vi "Aplicacao_v02.vi"() -> ()   [LabVIEW 2014]
uses:
  LabView_v03/testStateMachineCtr.ctl
  LabView_v03/testMachineCtr.ctl
  <vilib>/Analysis/baseanly.llb/Mean (DBL).vi
  <vilib>/express/express shared/transition.llb/Dynamic To Waveform Array.vi
  <vilib>/express/express signal manip/GetorSetDDTAttributes/Set DDT Attributes/SetT0.vi
  <vilib>/express/express shared/transition.llb/Waveform Array To Dynamic.vi
  <vilib>/express/express signal manip/GetorSetDDTAttributes/Set DDT Attributes/Set DDT Properties.xnode
  <vilib>/Analysis/NI_AALBase.lvlib
panel:
  in  "editSetPathToFile":path
  out "ledForce":bool caption="Célula de Carga"
  out "ledSpeed":bool caption="Velocidade"
  out "ledTempB":bool caption="Temperatura B"
  out "ledTempA":bool caption="Temperatura A"
  out "ledTempRef":bool caption="Referência"
  in  "buttonExit":bool
  in  "buttonStop":bool
  in  "buttonStart":bool
  out "graphForce":dynamicdata(graph)
  in  "editOffsetForce":dbl caption="Tara" min=0.0 max=100.0 step=0.1
  in  "editSetForce":dbl caption="Fator de conversão"
  out "editForce":dbl caption="Força (Kgf)" format="%#_4f"
  out "graphSpeed":dynamicdata(graph)
  in  "editSetSpeed":dbl caption="Fator de conversão"
  out "editSpeed":dbl caption="Velocidade (km/h)" format="%#_4f"
  out "editEngineSpeed":dbl caption="Rotação (RPM)" format="%#_4f"
  in  "buttonMotor":bool
  in  "buttonBrake":bool
  in  "editSetWaitLowerTime":u32 caption="Tempo de espera (s)"
  in  "editSetWaitUpperTime":u32 caption="Tempo de espera (s)"
  in  "editSetNumberOfCycles":u32 caption="Número de ciclos" max=999 step=1 format="%0d"
  in  "editSetLowerLimit":u32 caption="Limite inferior (km/h)"
  in  "editSetUpperLimit":u32 caption="Limite superior (km/h)"
  out "editTempB":dbl caption="Temperatura B (ºC)"
  out "editTempA":dbl caption="Temperatura A (ºC)"
  in  "editSetTempRef":dbl caption="Offset referência" step=0.01 format="%#_2f"
  out "editTempRef":dbl caption="Referência (ºC)"
  out "ledMotor":bool
  out "ledBrake":bool
  out "ledEnsaio":bool
  out "labelTotalCycle":string
  out "labelCurrentCycle":string
  out "error out":errorcluster
  out "labelSystemTitle":string
  in  "editCurrCycleCtr":u32
  in  "velocidade 2":u32
  out "velocidade":u32
  out "state":T1
  out "stateTest":T2
  # "Bancada de Frenagem - Ensaio"
  # "Sensores"
  # "Temperatura"
  # "Rotação"
  # "Célula de Carga"
  # "Configurações do ensaio"
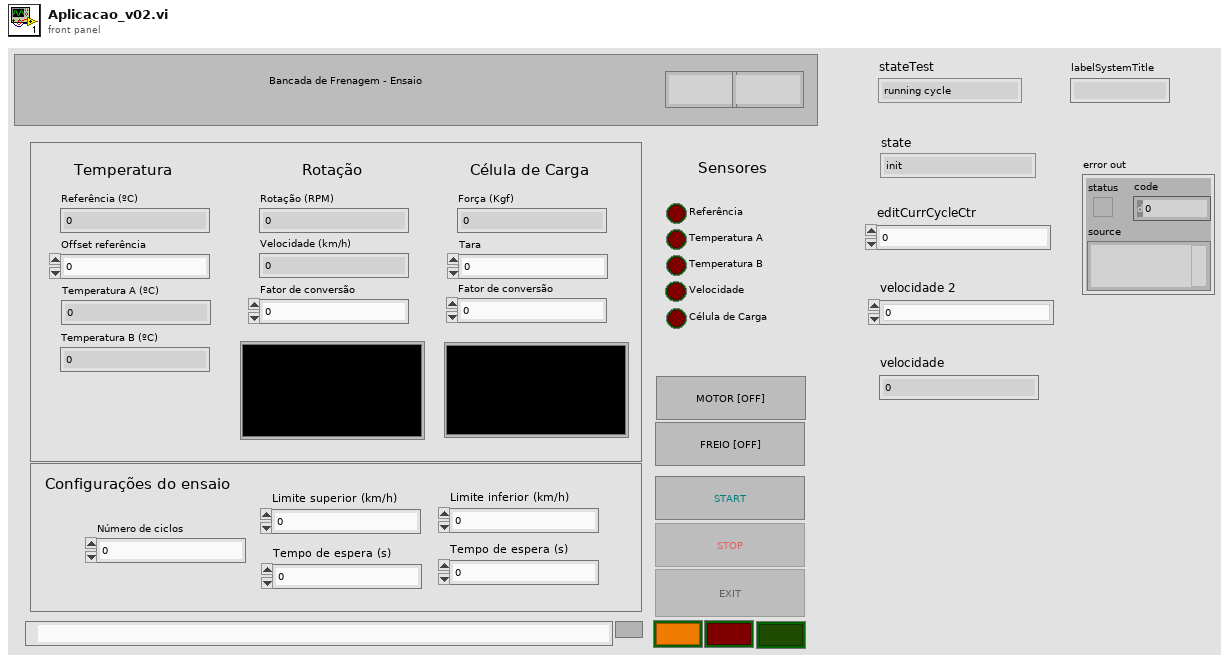
[diagram p1: front panel]
types:
  T1 = typedef "testMachineCtr.ctl" = enum16{"init", "ready", "running", "stopped", "finish", "shutdown"}
  T2 = typedef "testStateMachineCtr.ctl" = enum16{"running cycle", "acquiring data", "braking cycle", "stopping cycle"}
  T3 = enum8{"Enabled", "Disabled", "Disabled and Grayed Out"}
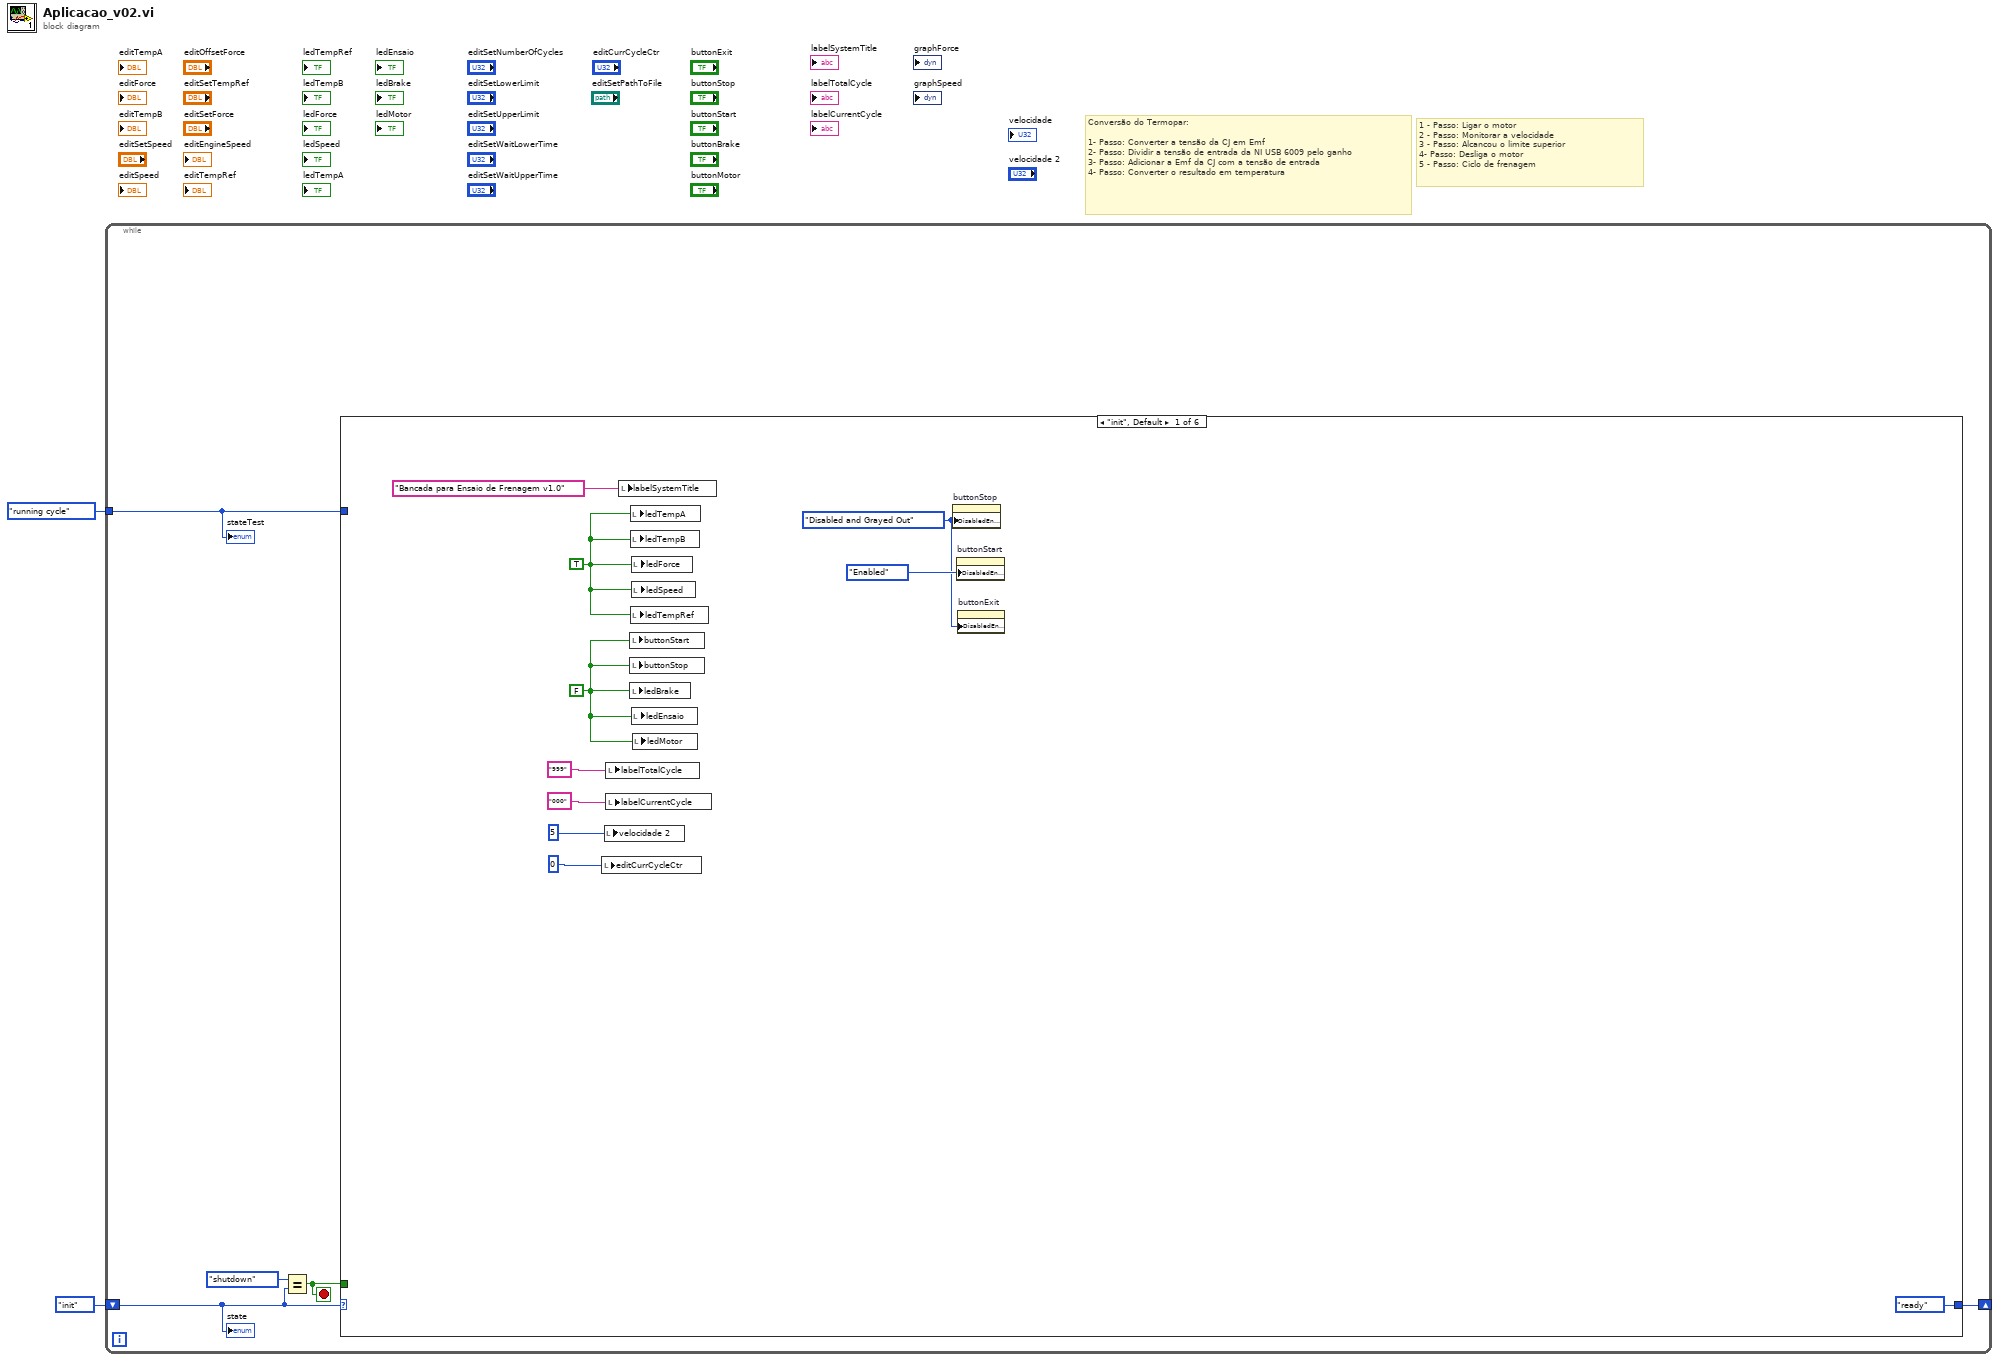
[diagram p0: block diagram]
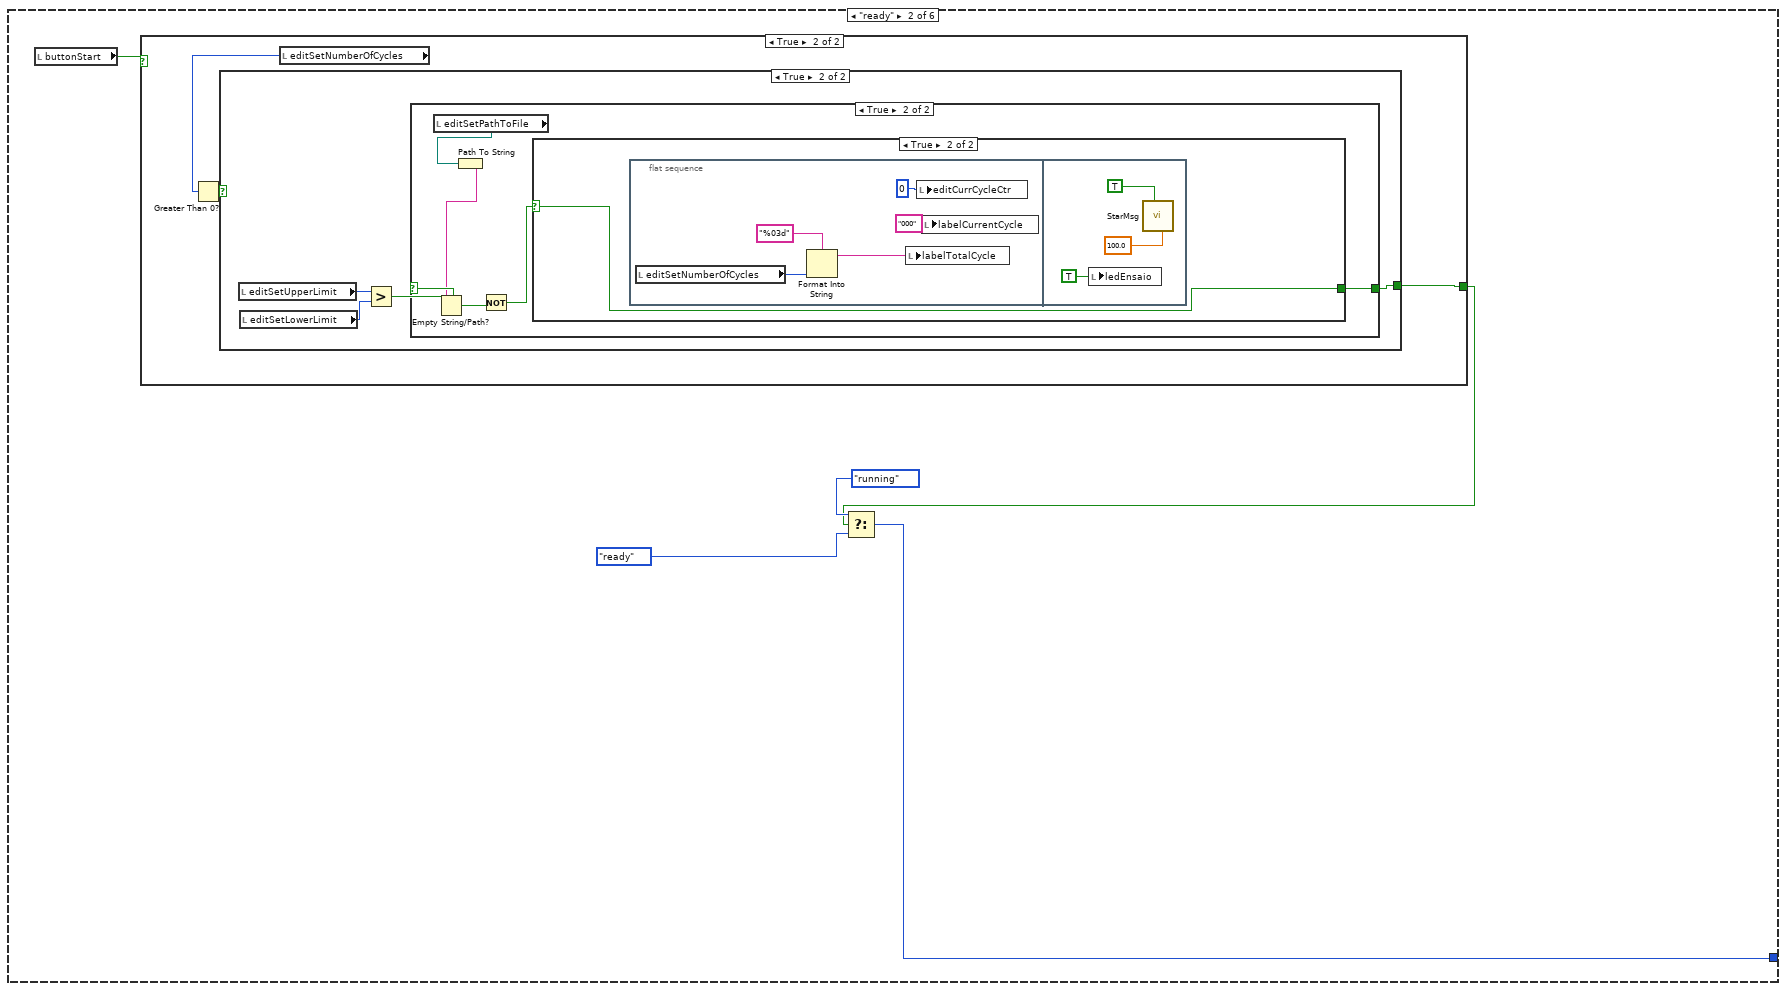
[diagram p2: hidden frame]
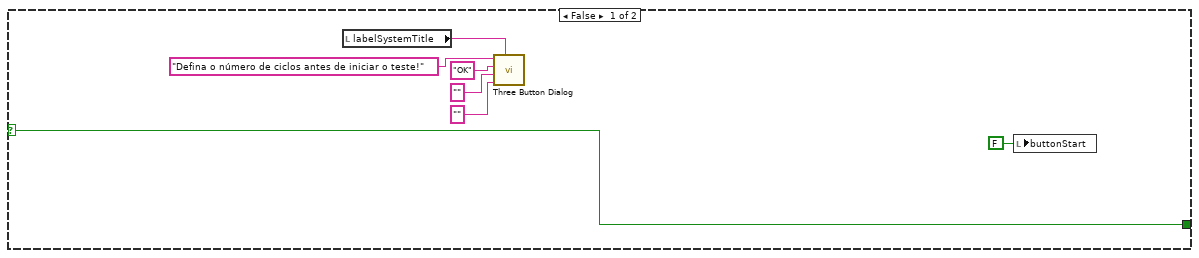
[diagram p4: hidden frame]
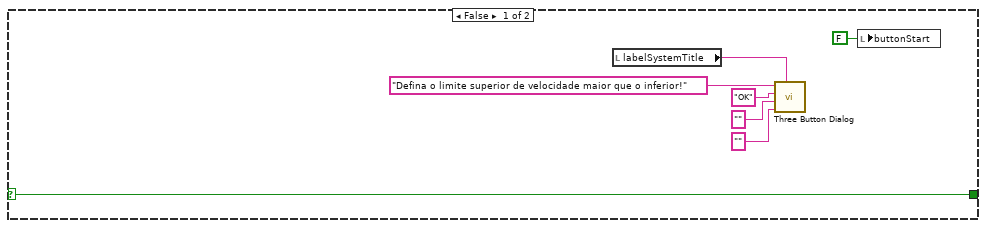
[diagram p5: hidden frame]
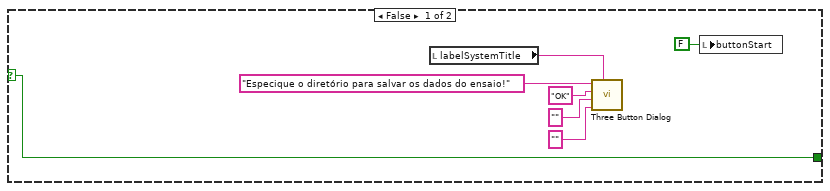
[diagram p6: hidden frame]
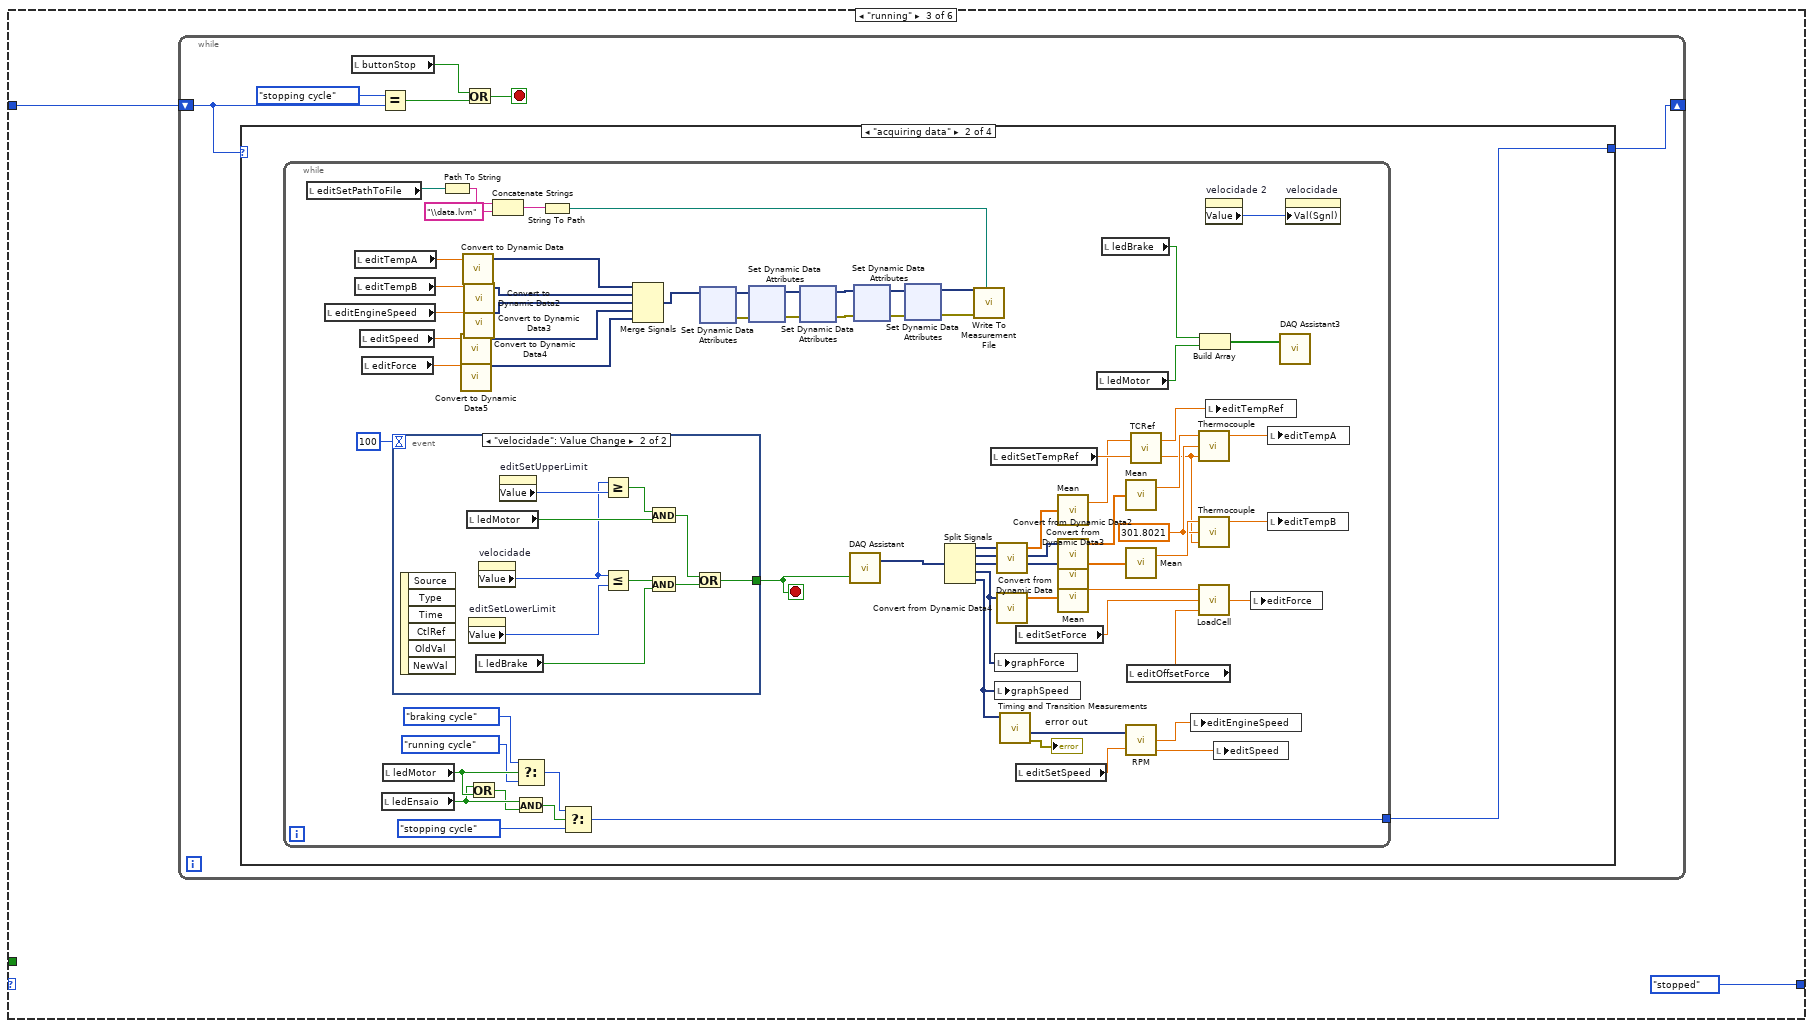
[diagram p7: hidden frame]
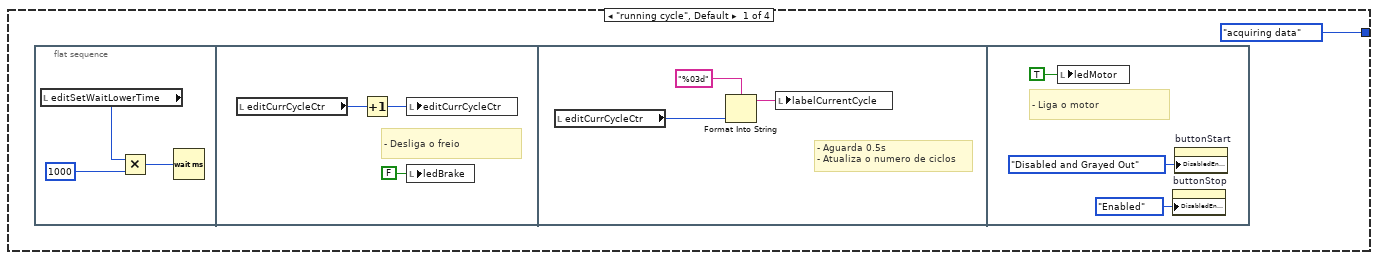
[diagram p8: hidden frame]
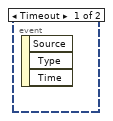
[diagram p9: hidden frame]
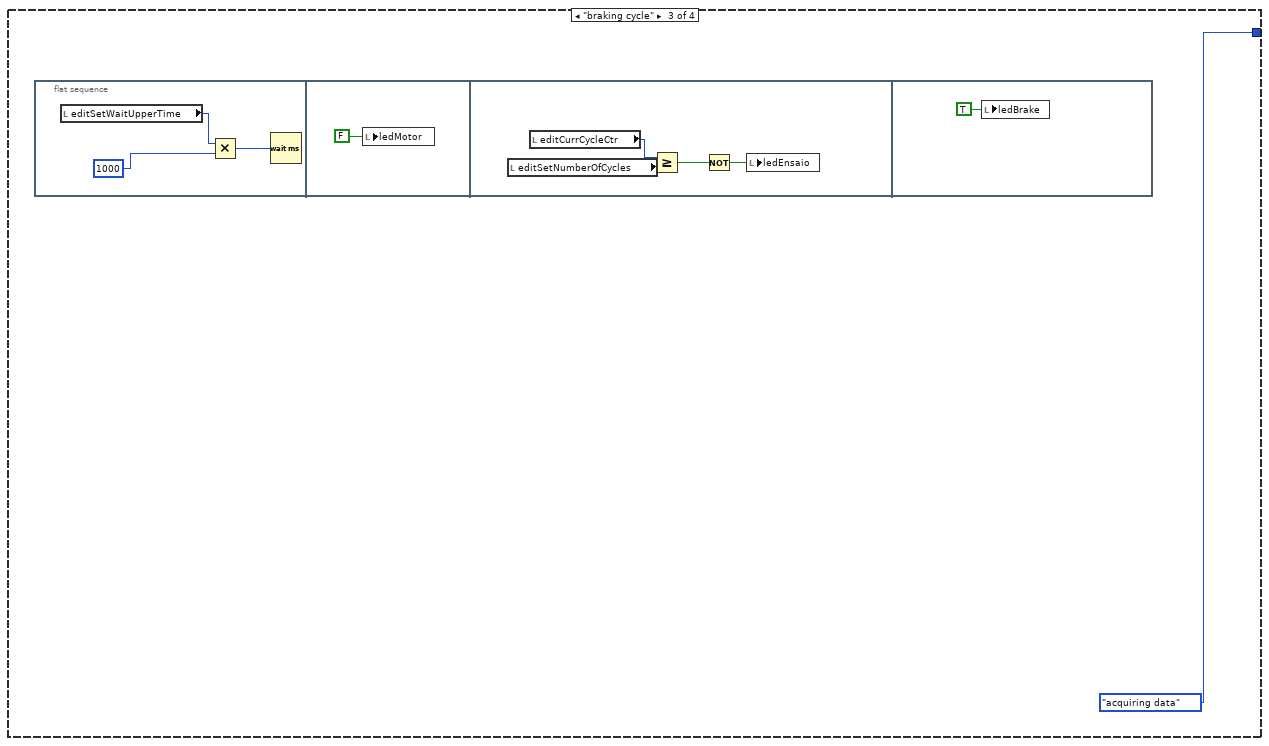
[diagram p10: hidden frame]
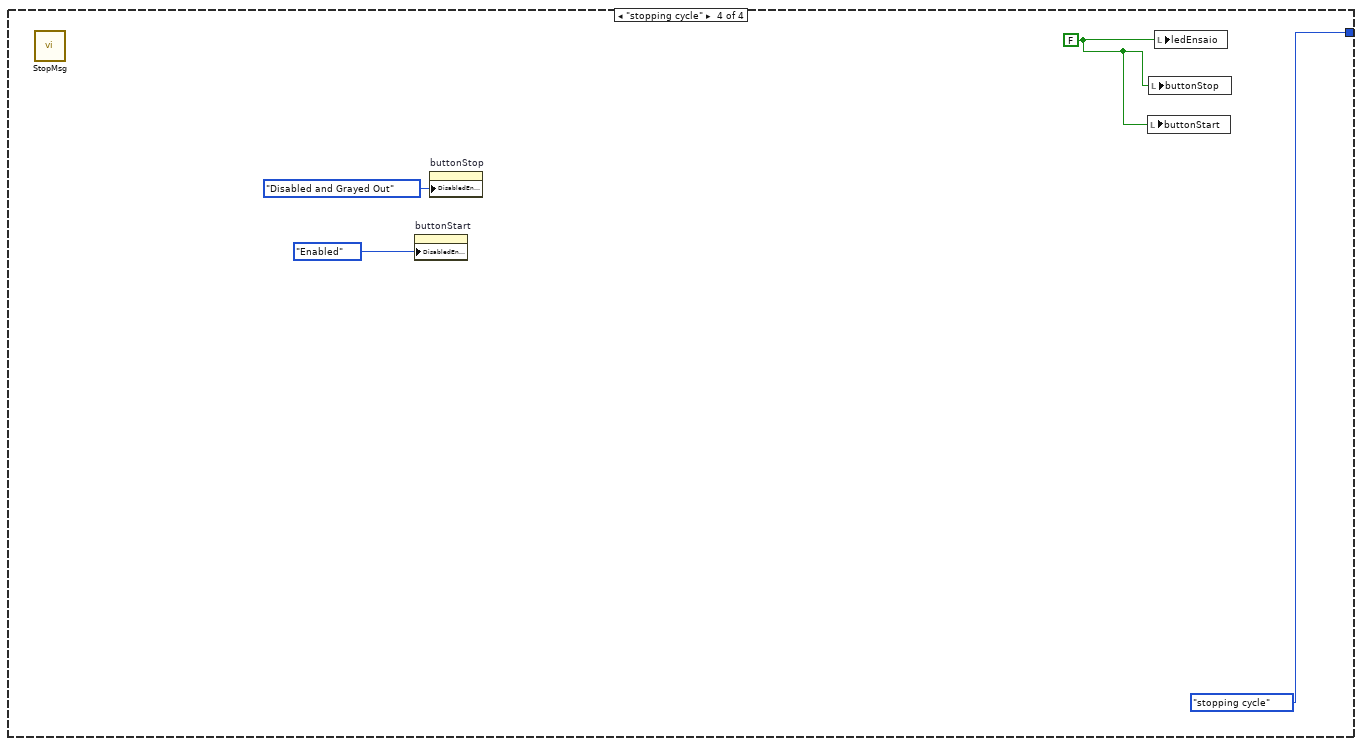
[diagram p11: hidden frame]
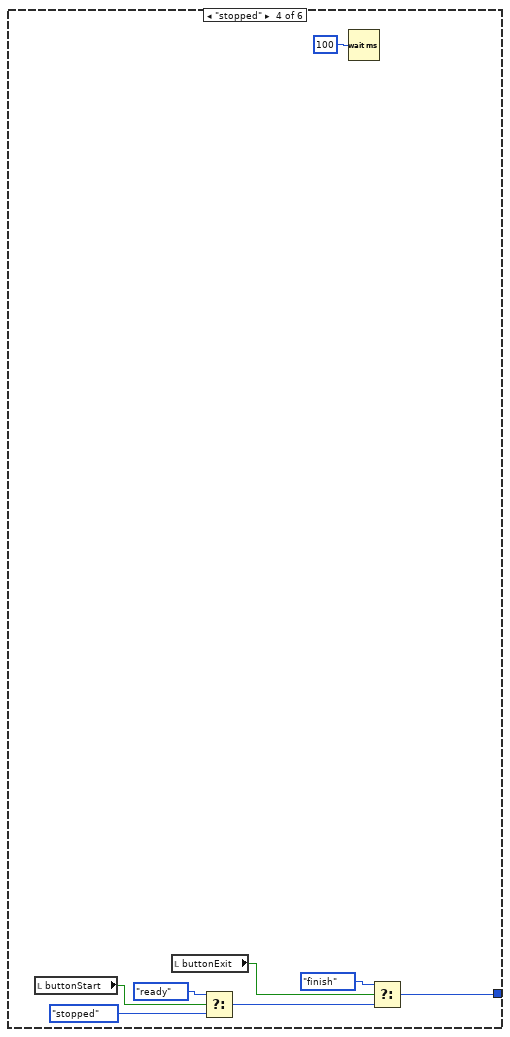
[diagram p12: hidden frame]
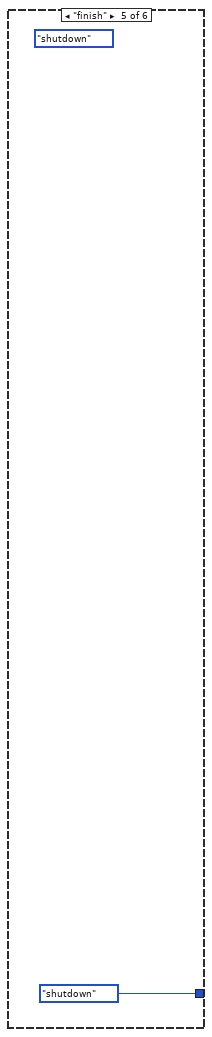
[diagram p13: hidden frame]
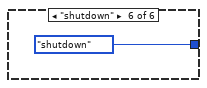
[diagram p14: hidden frame]
diagram:
  # "1 - Passo: Ligar o motor\n2 - Passo: Monitorar a velocidade\n3 - Passo: Alcancou o limite superior\n4- Passo: Desliga o motor\n5 - Passo: Ciclo de frenagem"
  # "Conversão do Termopar:\n\n1- Passo: Converter a tensão da CJ em Emf\n2- Passo: Dividir a tensão de entrada da NI USB 6009 pelo ganho\n3- Passo: Adicionar a Emf da CJ com a tensão de entrada\n4- Passo: Converter o resultado em temperatura"
  n1 = while {
    shift-right: [w5] -> _
    shift-left: testMachineCtr."init" ("state") -> [w7]
    tunnel: testStateMachineCtr."running cycle" ("stateTest") -> [w4]
    stop <- w3 stop-if-true
    n2 = Equal?(x=testMachineCtr."shutdown" ("state"), y=w7) -> (x = y?=w3:bool)
    n3 = case shown="\"init\", Default" w7 {
      tunnel: w3 -> [_ _ _ _ _ _]
      tunnel: [testMachineCtr."ready" ("state") w20 testMachineCtr."stopped" ("state") w275 testMachineCtr."shutdown" ("state") testMachineCtr."shutdown" ("state")] -> w5
      tunnel: w4 -> [_ _ w66 _ _ _]
      frame "init", Default {
        w8 = T3."Disabled and Grayed Out" ("Disabled")
        w10 = TRUE
        w15 = FALSE ("motor")
        n4 = local write "editCurrCycleCtr"(u32 0 ("currentCycleCtr")) -> ()
        n5 = local write "velocidade 2"(u32 5 ("velocidade 2")) -> ()
        n6 = local write "labelTotalCycle"("999" ("totalCycle")) -> ()
        n7 = local write "labelCurrentCycle"("000" ("currentCycle")) -> ()
        n8 = local write "labelSystemTitle"("Bancada para Ensaio de Frenagem v1.0" ("systemTitle")) -> ()
        n9 = local write "buttonStart"(w15) -> ()
        n10 = local write "buttonStop"(w15) -> ()
        n11 = local write "ledBrake"(w15) -> ()
        n12 = local write "ledTempA"(w10) -> ()
        n13 = local write "ledTempB"(w10) -> ()
        n14 = local write "ledTempRef"(w10) -> ()
        n15 = local write "ledForce"(w10) -> ()
        n16 = local write "ledSpeed"(w10) -> ()
        n17 = local write "ledEnsaio"(w15) -> ()
        n18 = local write "ledMotor"(w15) -> ()
        n19 = property on="buttonStop" class="Bool (strict)"("DisabledEnum"=w8) -> ()  [unwired: 2 in, 2 out]
        n20 = property on="buttonStart" class="Bool (strict)"("DisabledEnum"=T3."Enabled" ("Disabled")) -> ()  [unwired: 2 in, 2 out]
        n21 = property on="buttonExit" class="Bool (strict)"("DisabledEnum"=w8) -> ()  [unwired: 2 in, 2 out]
      }
      frame "ready" {
        n22 = local read "buttonStart"() -> (w19:bool)
        n23 = case shown="True" w19 {
          selector: w19 -> [w23 _]
          tunnel: [w23 w24] -> w18
          frame False {
          }
          frame True {
            n24 = local read "editSetNumberOfCycles"() -> (w26:u32)
            n25 = Greater Than 0?(x=w26) -> (x > 0?=w25:bool)
            n26 = case shown="True" w25 {
              selector: w25 -> [w33 _]
              tunnel: [w33 w34] -> w24
              frame False {
                n27 = local read "labelSystemTitle"() -> (w28:string)
                n28 = call <vilib>:"Three Button Dialog.vi"("Window Title (\"\")"=w28, "Right Button Text (\"Cancel\")"="" ("Right Button Text (\"Cancel\")"), "Center Button Text (\"No\")"="" ("Center Button Text (\"No\")"), "Left Button Text (\"Yes\")"="OK" ("Left Button Text (\"Yes\")"), "message"="Defina o número de ciclos antes de iniciar o teste!") -> ()  [unwired: 6 in, 1 out]
                n29 = local write "buttonStart"(FALSE ("startButton")) -> ()
              }
              frame True {
                n30 = local read "editSetUpperLimit"() -> (w36:u32)
                n31 = local read "editSetLowerLimit"() -> (w35:u32)
                n32 = Greater?(x=w36, y=w35) -> (0:w37:bool)
                n33 = case shown="True" w37 {
                  selector: w37 -> [w44 _]
                  tunnel: [w44 w47] -> w34
                  frame False {
                    n34 = local read "labelSystemTitle"() -> (w39:string)
                    n35 = call <vilib>:"Three Button Dialog.vi"("Window Title (\"\")"=w39, "Right Button Text (\"Cancel\")"="" ("Right Button Text (\"Cancel\")"), "Center Button Text (\"No\")"="" ("Center Button Text (\"No\")"), "Left Button Text (\"Yes\")"="OK" ("Left Button Text (\"Yes\")"), "message"="Defina o limite superior de velocidade maior que o inferior!") -> ()  [unwired: 6 in, 1 out]
                    n36 = local write "buttonStart"(FALSE ("startButton")) -> ()
                  }
                  frame True {
                    n37 = local read "editSetPathToFile"() -> (w49:path)
                    n38 = Path To String(path=w49) -> (string=w48:string)
                    n39 = Empty String/Path?(string/path=w48) -> (empty?=w46:bool)
                    n40 = Not(x=w46) -> (.not. x?=w45:bool)
                    n41 = case shown="True" w45 {
                      selector: w45 -> [w56 w57]
                      tunnel: [w56 w57] -> w47
                      frame False {
                        n42 = local read "labelSystemTitle"() -> (w51:string)
                        n43 = call <vilib>:"Three Button Dialog.vi"("Window Title (\"\")"=w51, "Right Button Text (\"Cancel\")"="" ("Right Button Text (\"Cancel\")"), "Center Button Text (\"No\")"="" ("Center Button Text (\"No\")"), "Left Button Text (\"Yes\")"="OK" ("Left Button Text (\"Yes\")"), "message"="Especique o diretório para salvar os dados do ensaio!") -> ()  [unwired: 6 in, 1 out]
                        n44 = local write "buttonStart"(FALSE ("startButton")) -> ()
                      }
                      frame True {
                        n45 = flat-sequence {
                          frame #0 {
                            n46 = local read "editSetNumberOfCycles"() -> (w60:u32)
                            n47 = Format Into String(format string="%03d", w60) -> (resulting string=w61:string)  [unwired: 2 in, 1 out]
                            n48 = local write "labelTotalCycle"(w61) -> ()
                            n49 = local write "editCurrCycleCtr"(u32 0 ("currentCycleCtr")) -> ()
                            n50 = local write "labelCurrentCycle"("000" ("currentCycle")) -> ()
                          }
                          frame #1 {
                            n51 = local write "ledEnsaio"(TRUE ("ensaio")) -> ()
                            n52 = call "StarMsg.vi"("Show"=TRUE, "Max Value (100)"=100.0) -> ()  [unwired: 7 in, 2 out]
                          }
                        }
                      }
                    }
                  }
                }
              }
            }
          }
        }
        n53 = Select(t=testMachineCtr."running" ("state"), s=w18, f=testMachineCtr."ready" ("state")) -> (s? t:f=w20:T1)
      }
      frame "running" {
        n54 = while {
          shift-right: [w72] -> _
          shift-left: w66 -> [w69]
          stop <- w68 stop-if-true
          n55 = case shown="\"acquiring data\"" w69 {
            tunnel: [testStateMachineCtr."acquiring data" ("stateTest") w87 testStateMachineCtr."acquiring data" ("stateTest") testStateMachineCtr."stopping cycle" ("stateTest")] -> w72
            frame "running cycle", Default {
              n56 = flat-sequence {
                frame #0 {
                  n57 = local read "editSetWaitLowerTime"() -> (w75:u32)
                  n58 = Multiply(x=w75, y=u32 1000 ("milliseconds to wait")) -> (x*y=w77:u32)
                  n59 = Wait (ms)(milliseconds to wait=w77) -> ()  [unwired: 1 out]
                }
                frame #1 {
                  # "- Desliga o freio"
                  n60 = local read "editCurrCycleCtr"() -> (w79:u32)
                  n61 = Increment(x=w79) -> (x+1=w78:u32)
                  n62 = local write "editCurrCycleCtr"(w78) -> ()
                  n63 = local write "ledBrake"(FALSE ("freio")) -> ()
                }
                frame #2 {
                  # "- Aguarda 0.5s \n- Atualiza o numero de ciclos"
                  n64 = local read "editCurrCycleCtr"() -> (w81:u32)
                  n65 = Format Into String(format string="%03d", w81) -> (resulting string=w82:string)  [unwired: 2 in, 1 out]
                  n66 = local write "labelCurrentCycle"(w82) -> ()
                }
                frame #3 {
                  # "- Liga o motor"
                  n67 = local write "ledMotor"(TRUE ("motor")) -> ()
                  n68 = property on="buttonStop" class="Bool (strict)"("DisabledEnum"=T3."Enabled" ("Disabled")) -> ()  [unwired: 2 in, 2 out]
                  n69 = property on="buttonStart" class="Bool (strict)"("DisabledEnum"=T3."Disabled and Grayed Out" ("Disabled")) -> ()  [unwired: 2 in, 2 out]
                }
              }
            }
            frame "acquiring data" {
              n70 = while {
                tunnel: [w149] -> w87
                stop <- w141 stop-if-true
                w130 = 301.8021 ("factor")
                n71 = local read "editSetPathToFile"() -> (w112:path)
                n72 = local read "editEngineSpeed"() -> (w97:dbl)
                n73 = local read "editTempA"() -> (w100:dbl)
                n74 = local read "editTempB"() -> (w98:dbl)
                n75 = local read "editSpeed"() -> (w96:dbl)
                n76 = local read "editForce"() -> (w95:dbl)
                n77 = local read "ledEnsaio"() -> (w152:bool)
                n78 = local read "ledMotor"() -> (w153:bool)
                n79 = event shown="[1] \"velocidade\": Value Change" {
                  selector: _ -> [_ _]
                  dyn-events: _ -> [_ _]
                  timeout: 100 -> [_ _]
                  tunnel: [_ w247] -> w141
                  event Timeout {
                    n80 = event-data() -> ()  [unwired: 1 in, 3 out]
                  }
                  event "velocidade": Value Change {
                    n81 = event-data() -> ()  [unwired: 1 in, 6 out]
                    n82 = local read "ledMotor"() -> (w254:bool)
                    n83 = property on="editSetLowerLimit" class="DigNum (strict)"() -> ("Value"=w252:u32)  [unwired: 2 in, 2 out]
                    n84 = local read "ledBrake"() -> (w251:bool)
                    n85 = property on="velocidade" class="DigNum (strict)"() -> ("Value"=w253:u32)  [unwired: 2 in, 2 out]
                    n86 = property on="editSetUpperLimit" class="DigNum (strict)"() -> ("Value"=w256:u32)  [unwired: 2 in, 2 out]
                    n87 = Greater Or Equal?(x=w253, y=w256) -> (x >= y?=w255:bool)
                    n88 = Less Or Equal?(x=w253, y=w252) -> (x <= y?=w250:bool)
                    n89 = And(x=w255, y=w254) -> (x .and. y?=w248:bool)
                    n90 = And(x=w250, y=w251) -> (x .and. y?=w249:bool)
                    n91 = Or(x=w248, y=w249) -> (x .or. y?=w247:bool)
                  }
                }
                n92 = Path To String(path=w112) -> (string=w113:string)
                n93 = call "Convert to Dynamic Data4"("Double"=w96) -> ("Dynamic Data Type"=w92:dynamicdata)  [unwired: 3 in]
                n94 = call "Convert to Dynamic Data5"("Double"=w95) -> ("Dynamic Data Type"=w91:dynamicdata)  [unwired: 3 in]
                n95 = call "Convert to Dynamic Data"("Double"=w100) -> ("Dynamic Data Type"=w99:dynamicdata)  [unwired: 3 in]
                n96 = call "Convert to Dynamic Data2"("Double"=w98) -> ("Dynamic Data Type"=w94:dynamicdata)  [unwired: 3 in]
                n97 = call "Convert to Dynamic Data3"("Double"=w97) -> ("Dynamic Data Type"=w93:dynamicdata)  [unwired: 3 in]
                n98 = Or(x=w152, y=w153) -> (x .or. y?=w151:bool)
                n99 = Concatenate Strings(w113, "\\data.lvm" ("string")) -> (w110:string)
                n100 = Select(t=testStateMachineCtr."braking cycle" ("stateTest"), s=w153, f=testStateMachineCtr."running cycle" ("stateTest")) -> (s? t:f=w154:T2)
                n101 = And(x=w152, y=w151) -> (x .and. y?=w150:bool)
                n102 = String To Path(string=w110) -> (path=w109:path)
                n103 = Select(t=w154, s=w150, f=testStateMachineCtr."stopping cycle" ("stateTest")) -> (s? t:f=w149:T2)
                n104 = Merge Signals(w99, w94, w93, w92, w91) -> (w90:dynamicdata)
                n105 = xnode ("Set Dynamic Data Attributes")("Signals In"=w90) -> ("Signals Out"=w108:dynamicdata, "error out"=w106:errorcluster)  [unwired: 4 in]
                n106 = xnode ("Set Dynamic Data Attributes")("Signals In"=w108, "error in"=w106) -> ("Signals Out"=w107:dynamicdata, "error out"=w105:errorcluster)  [unwired: 3 in]
                n107 = xnode ("Set Dynamic Data Attributes")("Signals In"=w107, "error in"=w105) -> ("Signals Out"=w89:dynamicdata, "error out"=w104:errorcluster)  [unwired: 3 in]
                n108 = call "DAQ Assistant"("stop (F)"=w141) -> ("data"=w145:dynamicdata)  [unwired: 15 in, 3 out]
                n109 = xnode ("Set Dynamic Data Attributes")("Signals In"=w89, "error in"=w104) -> ("Signals Out"=w88:dynamicdata, "error out"=w103:errorcluster)  [unwired: 3 in]
                n110 = xnode ("Set Dynamic Data Attributes")("Signals In"=w88, "error in"=w103) -> ("Signals Out"=w102:dynamicdata, "error out"=w101:errorcluster)  [unwired: 3 in]
                n111 = Split Signals(w145) -> (w142:dynamicdata, w134:dynamicdata, w136:dynamicdata, w124:dynamicdata, w125:dynamicdata)  [unwired: 5 in]
                n112 = call "Write To Measurement File"("Signals"=w102, "error in (no error)"=w101, "Filename"=w109) -> ()  [unwired: 14 in, 3 out]
                n113 = local read "editSetTempRef"() -> (w143:dbl)
                n114 = local write "graphForce"(w124) -> ()
                n115 = local write "graphSpeed"(w125) -> ()
                n116 = call "Convert from Dynamic Data"("Dynamic Data Type"=w142) -> ("Array"=w115:dbl[])  [unwired: 3 in]
                n117 = call "Convert from Dynamic Data4"("Dynamic Data Type"=w124) -> ("Array"=w133:dbl[])  [unwired: 3 in]
                n118 = call "Timing and Transition Measurements"("Signals"=w125) -> ("error out"=→"error out":errorcluster, "Frequency"=w122:dynamicdata)  [unwired: 9 in]
                n119 = local read "editSetForce"() -> (w117:dbl)
                n120 = local read "editSetSpeed"() -> (w121:dbl)
                n121 = call-poly <vilib>:"Mean.vi"("X"=w115) -> ("mean"=w114:dbl)  [unwired: 1 out]
                n122 = call "Convert from Dynamic Data2"("Dynamic Data Type"=w134) -> ("Array"=w137:dbl[])  [unwired: 3 in]
                n123 = call "Convert from Dynamic Data3"("Dynamic Data Type"=w136) -> ("Array"=w135:dbl[])  [unwired: 3 in]
                n124 = call-poly <vilib>:"Mean.vi"("X"=w133) -> ("mean"=w126:dbl)  [unwired: 1 out]
                n125 = local read "ledMotor"() -> (w138:bool)
                n126 = local read "ledBrake"() -> (w139:bool)
                n127 = call-poly <vilib>:"Mean.vi"("X"=w137) -> ("mean"=w132:dbl)  [unwired: 1 out]
                n128 = call-poly <vilib>:"Mean.vi"("X"=w135) -> ("mean"=w131:dbl)  [unwired: 1 out]
                n129 = call "RPM.vi"("data"=w122, "factor"=w121) -> ("RPM"=w119:dbl, "km/h"=w118:dbl)  [unwired: 1 out]
                n130 = local read "editOffsetForce"() -> (w116:dbl)
                n131 = call "TCRef.vi"("offset"=w143, "data"=w114) -> ("emf(mV)"=w129:dbl, "temp (degC)"=w144:dbl)
                n132 = local write "editEngineSpeed"(w119) -> ()
                n133 = call "Thermocouple.vi"("cj(mV)"=w129, "factor"=w130, "data"=w132) -> ("temp(degC)"=w128:dbl)  [unwired: 2 out]
                n134 = call "Thermocouple.vi"("cj(mV)"=w129, "factor"=w130, "data"=w131) -> ("temp(degC)"=w127:dbl)  [unwired: 2 out]
                n135 = call "LoadCell.vi"("tara"=w116, "factor"=w117, "data"=w126) -> ("force (Kgf)"=w120:dbl)
                n136 = Build Array(w139, w138) -> (w140:bool[])
                n137 = property on="velocidade 2" class="DigNum (strict)"() -> ("Value"=w155:u32)  [unwired: 2 in, 2 out]
                n138 = local write "editTempRef"(w144) -> ()
                n139 = local write "editSpeed"(w118) -> ()
                n140 = local write "editForce"(w120) -> ()
                n141 = local write "editTempA"(w128) -> ()
                n142 = local write "editTempB"(w127) -> ()
                n143 = call "DAQ Assistant3"("data"=w140) -> ()  [unwired: 17 in, 2 out]
                n144 = property on="velocidade" class="DigNum (strict)"("Val(Sgnl)"=w155) -> ()  [unwired: 2 in, 2 out]
              }
            }
            frame "braking cycle" {
              n145 = flat-sequence {
                frame #0 {
                  n146 = local read "editSetWaitUpperTime"() -> (w259:u32)
                  n147 = Multiply(x=w259, y=u32 1000) -> (x*y=w260:u32)
                  n148 = Wait (ms)(milliseconds to wait=w260) -> ()  [unwired: 1 out]
                }
                frame #1 {
                  n149 = local write "ledMotor"(FALSE ("motor")) -> ()
                }
                frame #2 {
                  n150 = local read "editSetNumberOfCycles"() -> (w264:u32)
                  n151 = local read "editCurrCycleCtr"() -> (w265:u32)
                  n152 = Greater Or Equal?(x=w265, y=w264) -> (x >= y?=w263:bool)
                  n153 = Not(x=w263) -> (.not. x?=w262:bool)
                  n154 = local write "ledEnsaio"(w262) -> ()
                }
                frame #3 {
                  n155 = local write "ledBrake"(TRUE ("freio")) -> ()
                }
              }
            }
            frame "stopping cycle" {
              w267 = FALSE ("ensaioLed")
              n156 = call "StopMsg.vi"() -> ()  [unwired: 9 in, 2 out]
              n157 = property on="buttonStart" class="Bool (strict)"("DisabledEnum"=T3."Enabled" ("Disabled")) -> ()  [unwired: 2 in, 2 out]
              n158 = property on="buttonStop" class="Bool (strict)"("DisabledEnum"=T3."Disabled and Grayed Out" ("Disabled")) -> ()  [unwired: 2 in, 2 out]
              n159 = local write "buttonStart"(w267) -> ()
              n160 = local write "buttonStop"(w267) -> ()
              n161 = local write "ledEnsaio"(w267) -> ()
            }
          }
          n162 = local read "buttonStop"() -> (w70:bool)
          n163 = Equal?(x=testStateMachineCtr."stopping cycle" ("stateTest"), y=w69) -> (x = y?=w71:bool)
          n164 = Or(x=w70, y=w71) -> (x .or. y?=w68:bool)
        }
      }
      frame "stopped" {
        n165 = local read "buttonStart"() -> (w276:bool)
        n166 = local read "buttonExit"() -> (w271:bool)
        n167 = Select(t=testMachineCtr."ready" ("state"), s=w276, f=testMachineCtr."stopped" ("state")) -> (s? t:f=w272:T1)
        n168 = Wait (ms)(milliseconds to wait=u32 100) -> ()  [unwired: 1 out]
        n169 = Select(t=testMachineCtr."finish" ("state"), s=w271, f=w272) -> (s? t:f=w275:T1)
      }
      frame "finish" {
        (unwired) testMachineCtr."shutdown" ("state")
      }
      frame "shutdown" {
      }
    }
    "state" <- w7
    "stateTest" <- w4
  }
